vi "MeasureRMS.vi"(0 "Sampling Rate":dbl, 1 "# of Samples":dbl) -> (7 "Waveform Graph":dynamicdata(graph), 8 "RMS":dbl)   [LabVIEW 2014]
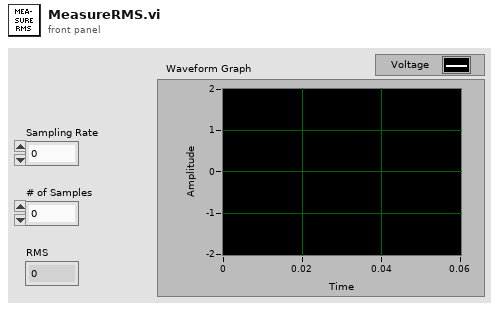
[diagram p1: front panel]
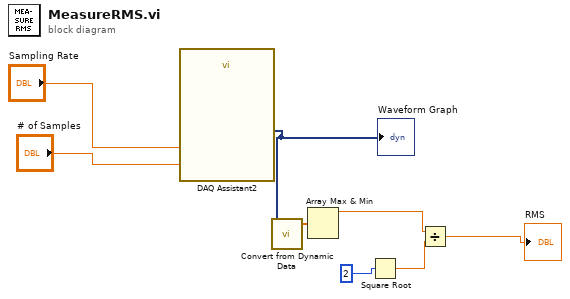
[diagram p0: block diagram]
diagram:
  n1 = call "DAQ Assistant2"("rate"="Sampling Rate", "number of samples"="# of Samples") -> ("data"=w6:dynamicdata)  [unwired: 15 in, 2 out]
  "Waveform Graph" <- w6
  n2 = call "Convert from Dynamic Data"("Dynamic Data Type"=w6) -> ("Array"=w5:dbl[])  [unwired: 3 in]
  n3 = Array Max & Min(array=w5) -> (max value=w3:dbl)  [unwired: 3 out]
  n4 = Square Root(x=2) -> (sqrt(x)=w4:dbl)
  n5 = Divide(x=w3, y=w4) -> (x/y=→"RMS":dbl)
